vi "Serie FIBONACCI.vi"() -> ()   [LabVIEW 2020]
panel:
  out "Array":i32[](array[numeric])
  in  "Cant. elementos":i32
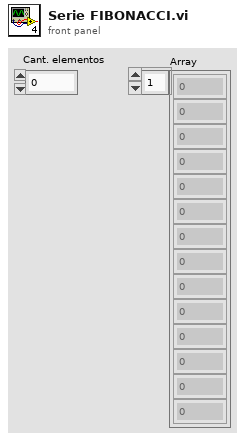
[diagram p1: front panel]
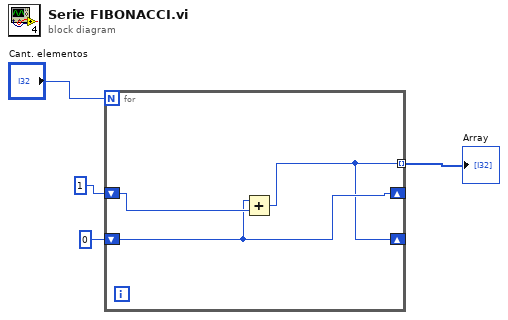
[diagram p0: block diagram]
diagram:
  n1 = for {
    N: "Cant. elementos" -> [_]
    shift-right: [w6] -> _
    shift-left: 1 -> [w7]
    shift-right: [w5] -> _
    shift-left: 0 -> [w6]
    tunnel: [w5] -> w1 mode=indexing
    n2 = Add(x=w6, y=w7) -> (x+y=w5:i32)
  }
  "Array" <- w1
